vi "Untitled 10 (SubVI).vi"(10 "Boolean 2":bool, 11 "Boolean":bool) -> (2 "carry":bool, 3 "sum":bool)   [LabVIEW 2015]
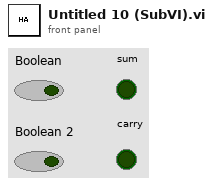
[diagram p1: front panel]
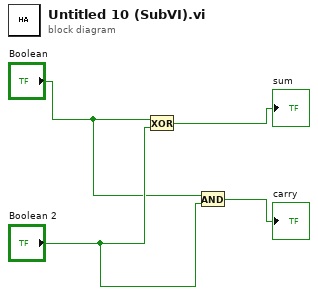
[diagram p0: block diagram]
diagram:
  n1 = Exclusive Or(1:"Boolean 2", 2:"Boolean") -> (0:→"sum":bool)
  n2 = And(x="Boolean", y="Boolean 2") -> (x .and. y?=→"carry":bool)
